vi "CCSA RPJ SLJC PF SubVI002.vi"(2 "Patrón original":T1, 3 "Toma original":T1) -> (0 "Toma original":T1(plugin-control), 1 "Patron rotado":T1(plugin-control) caption="Patrón rotado")   [LabVIEW 2021]
doc: "Rota una imagen con respeco a otra a partir de sus centroides"
uses:
  <vilib>/vision/Image Controls.llb/IMAQ Image.ctl
  <vilib>/vision/NI_Vision_Development_Module.lvlib
panel:
  out "Angle (deg)":dbl format="%.2f"
  out "Patrón original":T1(plugin-control)
  # "CUEVAS CERÓN SERGIO ALBERTO\nREYES PÉREZ JAVIER\nSALCEDO LICEA JUAN CARLOS"
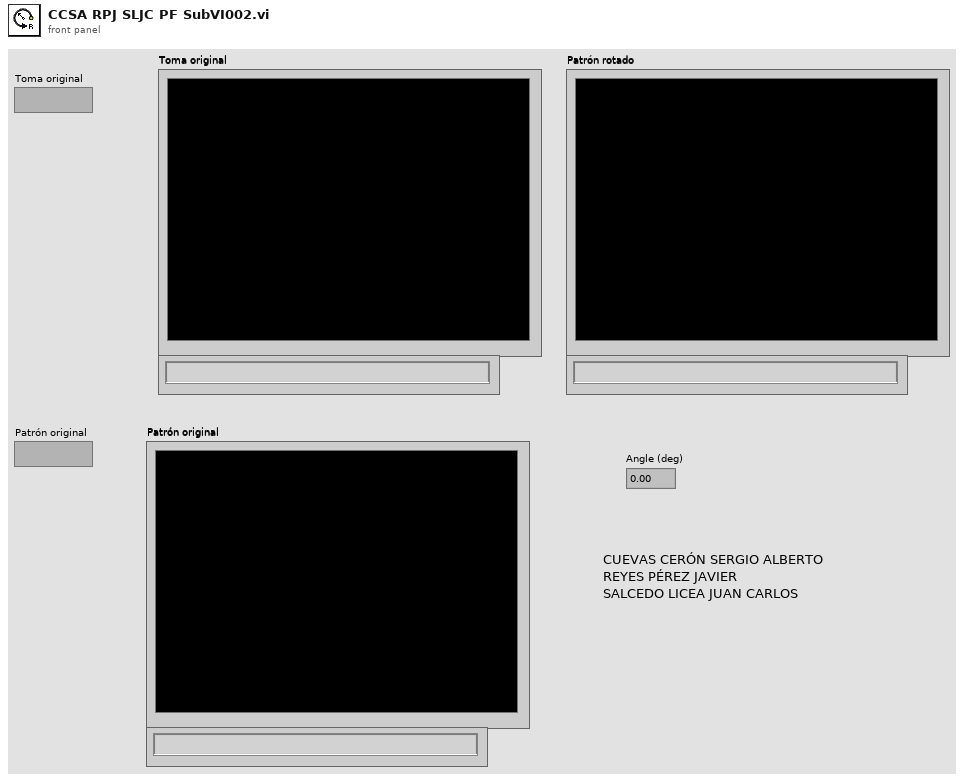
[diagram p1: front panel]
types:
  T1 = typedef "IMAQ Image.ctl" = refnum<image>
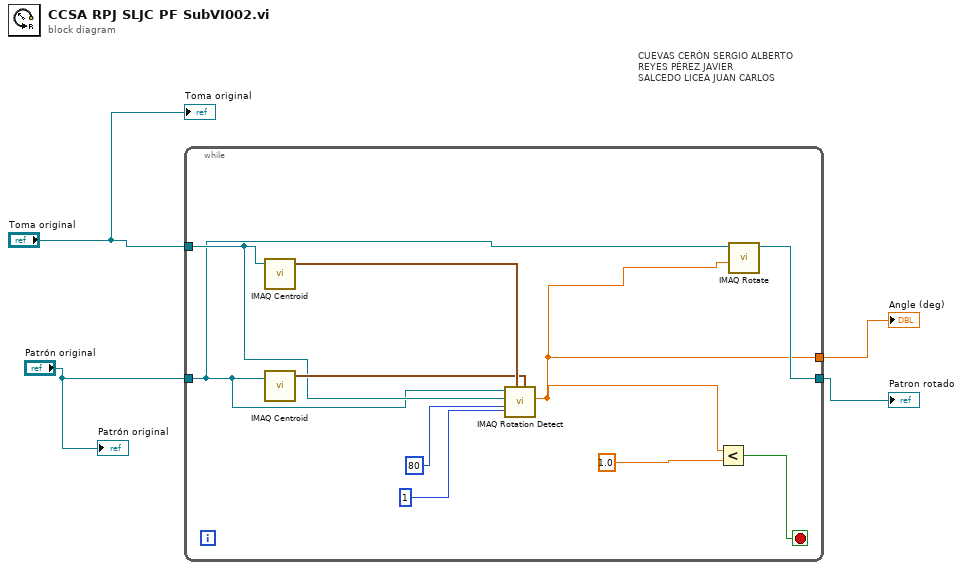
[diagram p0: block diagram]
diagram:
  # "CUEVAS CERÓN SERGIO ALBERTO\nREYES PÉREZ JAVIER\nSALCEDO LICEA JUAN CARLOS"
  n1 = while {
    tunnel: [w9] -> w3
    tunnel: "Toma original" -> [w6]
    tunnel: "Patrón original" -> [w5]
    tunnel: [w12] -> w4
    stop <- w10 stop-if-true
    n2 = call "IMAQ Centroid"("Image"=w6) -> ("Centroid"=w8:cluster{"X Centroid":sgl, "Y Centroid":sgl})  [unwired: 3 in, 1 out]
    n3 = call "IMAQ Centroid"("Image"=w5) -> ("Centroid"=w7:cluster{"X Centroid":sgl, "Y Centroid":sgl})  [unwired: 3 in, 1 out]
    n4 = call "IMAQ Rotation Detect"("Reference Center"=w7, "Precision (degrees)"=1, "Image 2 Center"=w8, "Radius"=80, "Image 2"=w6, "Reference Image"=w5) -> ("Angle (deg)"=w9:dbl)  [unwired: 3 in, 2 out]
    n5 = Less?(x=w9, y=1.0) -> (x < y?=w10:bool)
    n6 = call "IMAQ Rotate"("Angle (degrees)"=w9, "Image Src"=w5) -> ("Image Dst Out"=w12:T1)  [unwired: 8 in, 1 out]
  }
  "Patron rotado" <- w4
  "Angle (deg)" <- w3
  "Patrón original" <- "Patrón original"
  "Toma original" <- "Toma original"
